vi "Tecan_send_cmd.vi"() -> ()   [LabVIEW 2014]
uses:
  Project5_FISH_02/device/device_global.vi
  Project5_FISH_02/device/CAVRO_XC.llb/XC3P.lvclass
panel:
  in  "Command":string="O"
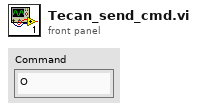
[diagram p1: front panel]
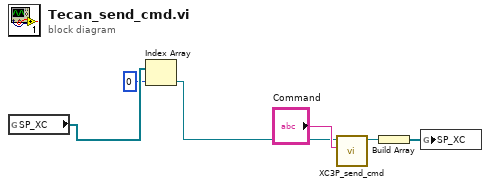
[diagram p0: block diagram]
diagram:
  n1 = global read "device_global.vi" "SP_XC"() -> (w3:refnum<class "XC3P.lvclass">[])
  n2 = Index Array(array=w3, index=0) -> (element=w1:refnum<class "XC3P.lvclass">)
  n3 = call-dynamic "XC3P_send_cmd.vi"("Command"="Command", "XC3P in"=w1) -> ("XC3P out"=w4:refnum<class "XC3P.lvclass">)  [unwired: 6 in, 3 out]
  n4 = Build Array(w4) -> (w5:refnum<class "XC3P.lvclass">[])
  n5 = global write "device_global.vi" "SP_XC"(w5) -> ()
